vi "Update FPGA Setup Data.vi"(8 "error in (no error)":errorcluster, 9 "FPGA Setup Parameters":T1={"FPGA Timing Constraints"={"frame.length Min"=530, "frame.ST_OFF Min"=15, "frame.ST_ON Min"=8, "frame.first data idx"=14, "frame.integ Offset"=6, "frame.integ Delay"=3, "frame.ad_latch Delay"=11, "frame.trig time Max"=0}, "FPGA Timing Ctrl"={"trig.time"=220, "integ.count 1"=400, "integ.count 2"=350, "encdr.latch ctrl"=1, "pixel.read count"=512, "clock.select"=2, "ad.clock offset"=16, "data.control reg"=2}, "FPGA Laser Config"={"laser.gain"=10, "laser.threshold Low"=1400, "laser.threshold High"=1900, "laser.dac init"=912, "laser.dac Min"=800, "laser.dac Max"=4000, "laser.config reg"=3}, "FPGA Peak Proc Cfg"={"PD.threshold"=0, "PD.width detect Min"=0, "PD.sensor pixels"=512, "PD.config reg"=23}, "FPGA SPI Cfg"={"SPI Divide Value"=1, "SPI config reg"=1}} {"FPGA SPI Cfg"."SPI config reg" format="%03b"; "FPGA Peak Proc Cfg"."PD.config reg" format="%05b"; "FPGA Laser Config"."laser.config reg" format="%02b"; "FPGA Timing Ctrl"."data.control reg" format="%03b"; "FPGA Timing Constraints"."frame.trig time Max" format="%0.0f"}, 10 "Commit":bool) -> (0 "error out":errorcluster)   [LabVIEW 2015, in "Tool Module.lvlib"]
doc: "Updates the FPGA Setup Data in either the Tool working copy or as well to the Tool File non-volitile File System (if Commit==T).\n_____\nCreated using Delacor QMH Event Scripter 4.2.1.88."
uses:
  Tool Module.lvlib
  Tool Typedefs/_FPGA Setup Params Cluster--typedef.ctl
  Tool Typedefs/_FPGA Timing Constraints Cluster--typedef.ctl
  Tool Typedefs/_FPGA Timing Ctrl Cluster--typedef.ctl
  Tool Typedefs/_FPGA Laser Config Cluster--typedef.ctl
  Tool Typedefs/_FPGA Peak Proc Cfg Cluster--typedef.ctl
  Tool Typedefs/_FPGA SPI Cfg Cluster--typedef.ctl
  Update FPGA Setup Data Argument--cluster.ctl
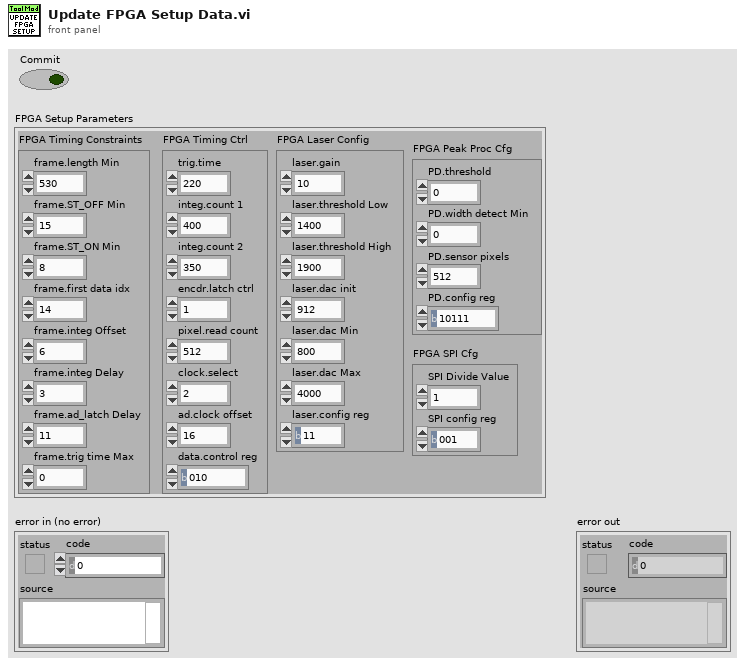
[diagram p1: front panel]
types:
  T1 = typedef "_FPGA Setup Params Cluster--typedef.ctl" = cluster{"FPGA Timing Constraints":T2, "FPGA Timing Ctrl":T3, "FPGA Laser Config":T4, "FPGA Peak Proc Cfg":T5, "FPGA SPI Cfg":T6}
  T2 = typedef "_FPGA Timing Constraints Cluster--typedef.ctl" = cluster{"frame.length Min":u16, "frame.ST_OFF Min":u16, "frame.ST_ON Min":u16, "frame.first data idx":u16, "frame.integ Offset":u16, "frame.integ Delay":u16, "frame.ad_latch Delay":u16, "frame.trig time Max":u32}
  T3 = typedef "_FPGA Timing Ctrl Cluster--typedef.ctl" = cluster{"trig.time":u32, "integ.count 1":u32, "integ.count 2":u32, "encdr.latch ctrl":u32, "pixel.read count":u16, "clock.select":u16, "ad.clock offset":u16, "data.control reg":u16}
  T4 = typedef "_FPGA Laser Config Cluster--typedef.ctl" = cluster{"laser.gain":i16, "laser.threshold Low":u16, "laser.threshold High":u16, "laser.dac init":u16, "laser.dac Min":u16, "laser.dac Max":u16, "laser.config reg":u16}
  T5 = typedef "_FPGA Peak Proc Cfg Cluster--typedef.ctl" = cluster{"PD.threshold":u16, "PD.width detect Min":u8, "PD.sensor pixels":u16, "PD.config reg":u16}
  T6 = typedef "_FPGA SPI Cfg Cluster--typedef.ctl" = cluster{"SPI Divide Value":u8, "SPI config reg":u16}
  T7 = typedef "Tool Module.lvlib/Update FPGA Setup Data Argument--cluster.ctl" = cluster{"Commit":bool, "FPGA Setup Parameters":T1}
  T8 = typedef "Tool Module.lvlib/Request Events--cluster.ctl" = cluster{"Stop Module":refnum<user-event>, "Show Panel":refnum<user-event>, "Hide Panel":refnum<user-event>, "Get Module Execution Status":refnum<user-event>, "Show Diagram":refnum<user-event>, "Test Trig 2":refnum<user-event>, "GOTO":refnum<user-event>, "Start Inspect":refnum<user-event>, "CONNECT":refnum<user-event>, "Get All Inspect Data":refnum<user-event>, "Get Inspection Limits":refnum<user-event>, "Set Inspection Limits":refnum<user-event>, "Update Status":refnum<user-event>, "Start Data Monitor":refnum<user-event>, "Get FPGA Setup Params":refnum<user-event>, "Set FPGA Setup Params":refnum<user-event>, "Set Tool Config":refnum<user-event>, "Get Tool Config":refnum<user-event>, "Set Integration Count":refnum<user-event>, "Set Laser Params":refnum<user-event>, "Get Mtrl Ctrl Reg":refnum<user-event>, "Commit Ctrl Reg":refnum<user-event>, "Set Event Logger":refnum<user-event>, "Write to File":refnum<user-event>, "Read from File":refnum<user-event>, "Set Device Temp Thresholds":refnum<user-event>, "Get Cycle Count":refnum<user-event>, "Return FPGA Setup Data":refnum<user-event>, "Update FPGA Setup Data":refnum<user-event>}
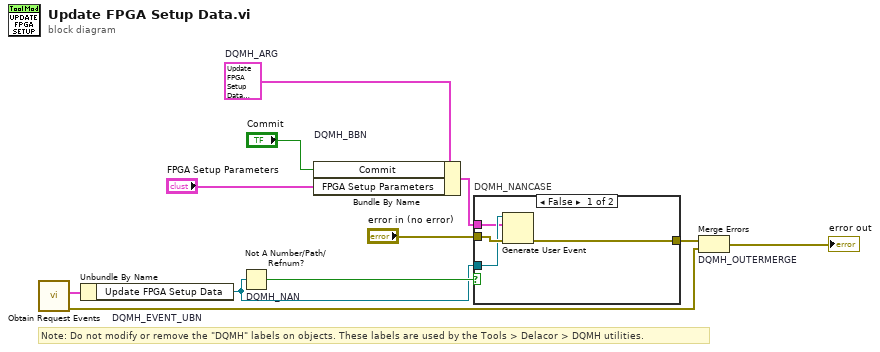
[diagram p0: block diagram]
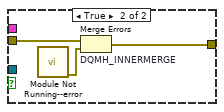
[diagram p2: hidden frame]
diagram:
  w5 = T7 {"Commit"=FALSE, "FPGA Setup Parameters"={"FPGA Timing Constraints"={"frame.length Min"=530, "frame.ST_OFF Min"=15, "frame.ST_ON Min"=8, "frame.first data idx"=14, "frame.integ Offset"=6, "frame.integ Delay"=3, "frame.ad_latch Delay"=11, "frame.trig time Max"=0}, "FPGA Timing Ctrl"={"trig.time"=220, "integ.count 1"=400, "integ.count 2"=350, "encdr.latch ctrl"=1, "pixel.read count"=512, "clock.select"=2, "ad.clock offset"=16, "data.control reg"=2}, "FPGA Laser Config"={"laser.gain"=10, "laser.threshold Low"=1400, "laser.threshold High"=1900, "laser.dac init"=912, "laser.dac Min"=800, "laser.dac Max"=4000, "laser.config reg"=3}, "FPGA Peak Proc Cfg"={"PD.threshold"=0, "PD.width detect Min"=0, "PD.sensor pixels"=512, "PD.config reg"=23}, "FPGA SPI Cfg"={"SPI Divide Value"=1, "SPI config reg"=1}}}  # DQMH_ARG
  # "Note: Do not modify or remove the \"DQMH\" labels on objects. These labels are used by the Tools > Delacor > DQMH utilities."
  n1 = call "Obtain Request Events.vi"() -> ("error out"=w2:errorcluster, "Tool Module Request Events"=w1:T8)  [unwired: 10 in]
  n2 = Unbundle By Name "DQMH_EVENT_UBN"(w1) -> ("Update FPGA Setup Data"=w7:refnum<user-event>)
  n3 = Not A Number/Path/Refnum? "DQMH_NAN"(number/path/refnum=w7) -> (NaN/Path/Refnum?=w8:bool)
  n4 = Bundle By Name "DQMH_BBN"(cluster=w5, "Commit"="Commit", "FPGA Setup Parameters"="FPGA Setup Parameters") -> (w9:T7)
  n5 = case "DQMH_NANCASE" shown="False" w8 {
    tunnel: "error in (no error)" -> [w15 w18]
    tunnel: [w14 w17] -> w6
    tunnel: w7 -> [w13 _]
    tunnel: w9 -> [w12 _]
    frame False {
      n6 = Generate User Event(user event=w13, event data cluster=w12, error in=w15) -> (error out=w14:errorcluster)  [unwired: 1 in, 1 out]
    }
    frame True {
      n7 = call "Module Not Running--error.vi"() -> ("error out"=w16:errorcluster)  [unwired: 11 in]
      n8 = Merge Errors "DQMH_INNERMERGE"(w18, w16) -> (w17:errorcluster)
    }
  }
  n9 = Merge Errors "DQMH_OUTERMERGE"(w6, w2) -> (→"error out":errorcluster)
